vi "Make Scaling param.vi"(0 "String (\"\")":string, 5 "Scaling":T1={"Floating Point Position (2)"=2, "Lower Scaling (0)"=0.0, "Upper Scaling (10000)"=100.0, "Unit Character (\"\")"=""} {"Floating Point Position (2)" min=0 max=5 step=1}, 11 "error in (no error)":errorcluster) -> (4 "String After":string, 15 "error out":errorcluster)   [LabVIEW 2020, in "Yokogawa GX Series.lvlib"]
doc: "This VI gets scaling parameter string and concat after input string."
uses:
  <instrlib>/Yokogawa GX Series/Yokogawa GX Series.lvlib
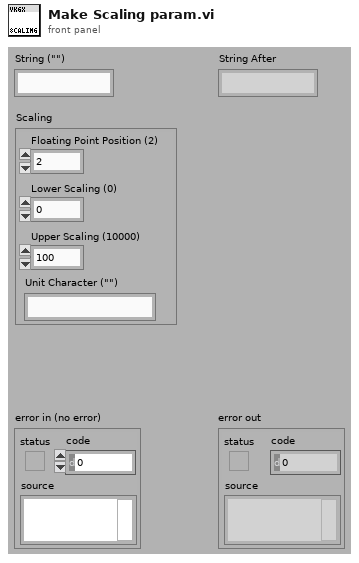
[diagram p1: front panel]
types:
  T1 = cluster{"Floating Point Position (2)":i32, "Lower Scaling (0)":dbl, "Upper Scaling (10000)":dbl, "Unit Character (\"\")":string}
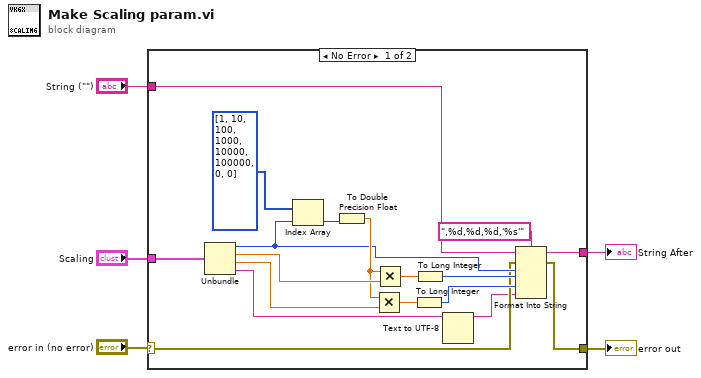
[diagram p0: block diagram]
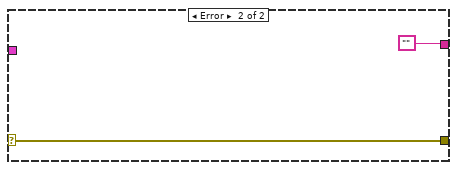
[diagram p2: hidden frame]
diagram:
  n1 = case shown="No Error" "error in (no error)" {
    selector: "error in (no error)" -> [w8 w24]
    tunnel: "Scaling" -> [w21 _]
    tunnel: [w15 ""] -> w4
    tunnel: [w10 w24] -> w3
    tunnel: "String (\"\")" -> [w9 _]
    frame No Error {
      n2 = Unbundle(w21) -> ("Floating Point Position (2)"=w13:i32, "Lower Scaling (0)"=w20:dbl, "Upper Scaling (10000)"=w18:dbl, "Unit Character (\"\")"=w7:string)
      n3 = Index Array(array=i32[] [1, 10, 100, 1000, 10000, 100000, 0, 0], index=w13) -> (element=w22:i32)
      n4 = To Double Precision Float(number=w22) -> (double precision float=w19:dbl)
      n5 = Multiply(x=w19, y=w18) -> (x*y=w16:dbl)
      n6 = Multiply(x=w19, y=w20) -> (x*y=w17:dbl)
      n7 = To Long Integer(number=w16) -> (32bit integer=w11:i32)
      n8 = To Long Integer(number=w17) -> (32bit integer=w12:i32)
      n9 = Text to UTF-8(11:w7) -> (3:w6:string)  [unwired: 2 in, 1 out]
      n10 = Format Into String(format string=",%d,%d,%d,'%s'", initial string=w9, error in=w8, w13, w12, w11, w6) -> (resulting string=w15:string, error out=w10:errorcluster)
    }
    frame Error {
    }
  }
  "error out" <- w3
  "String After" <- w4
